vi "BM0211-Image Editing.vi"(8 "error IN":errorcluster) -> (0 "error out":errorcluster)   [LabVIEW 2015]
uses:
  <vilib>/Utility/miscctls.llb/LVBoundsTypeDef.ctl
  <vilib>/Utility/miscctls.llb/LVPointTypeDef.ctl
  Galobal variable_TI.vi
panel:
  in  "Numeric":dbl
  out "2D Picture 2":picture
  out "Assembly ST-1":picture
  out "filenames":string[](array[string])
  out "selected path":path
  out "Boolean":bool
  in  "Vertical position":sgl(slide) min=-2000 max=2000 scale=-1000.0..2000.0 scale format="%#.0f"
  out "Horizontal position":sgl(slide) min=-2000 max=2000 scale=-1000.0..2000.0 scale format="%#.0f"
  in  "Zoom Factor":sgl(slide)=1.0 min=1 max=100 scale=0.0..200.0 scale format="%#.0f"
  out "2D Picture":picture
  in  "Stop Button":bool
  in  "Select Part":u16(ring) items=["P1.JPG", "P2.JPG", "P3.JPG", "P4.JPG", "P5.JPG", "P6.JPG", "P7.JPG", "P8.JPG", "P9.JPG", "P10.JPG", "P11.JPG", "P12.JPG", "P13.JPG", "P14.JPG", "P15.JPG", "P16.JPG", "P17.JPG"]
  in  "Save":bool
  in  "Select New":bool
  # "Image Editing"
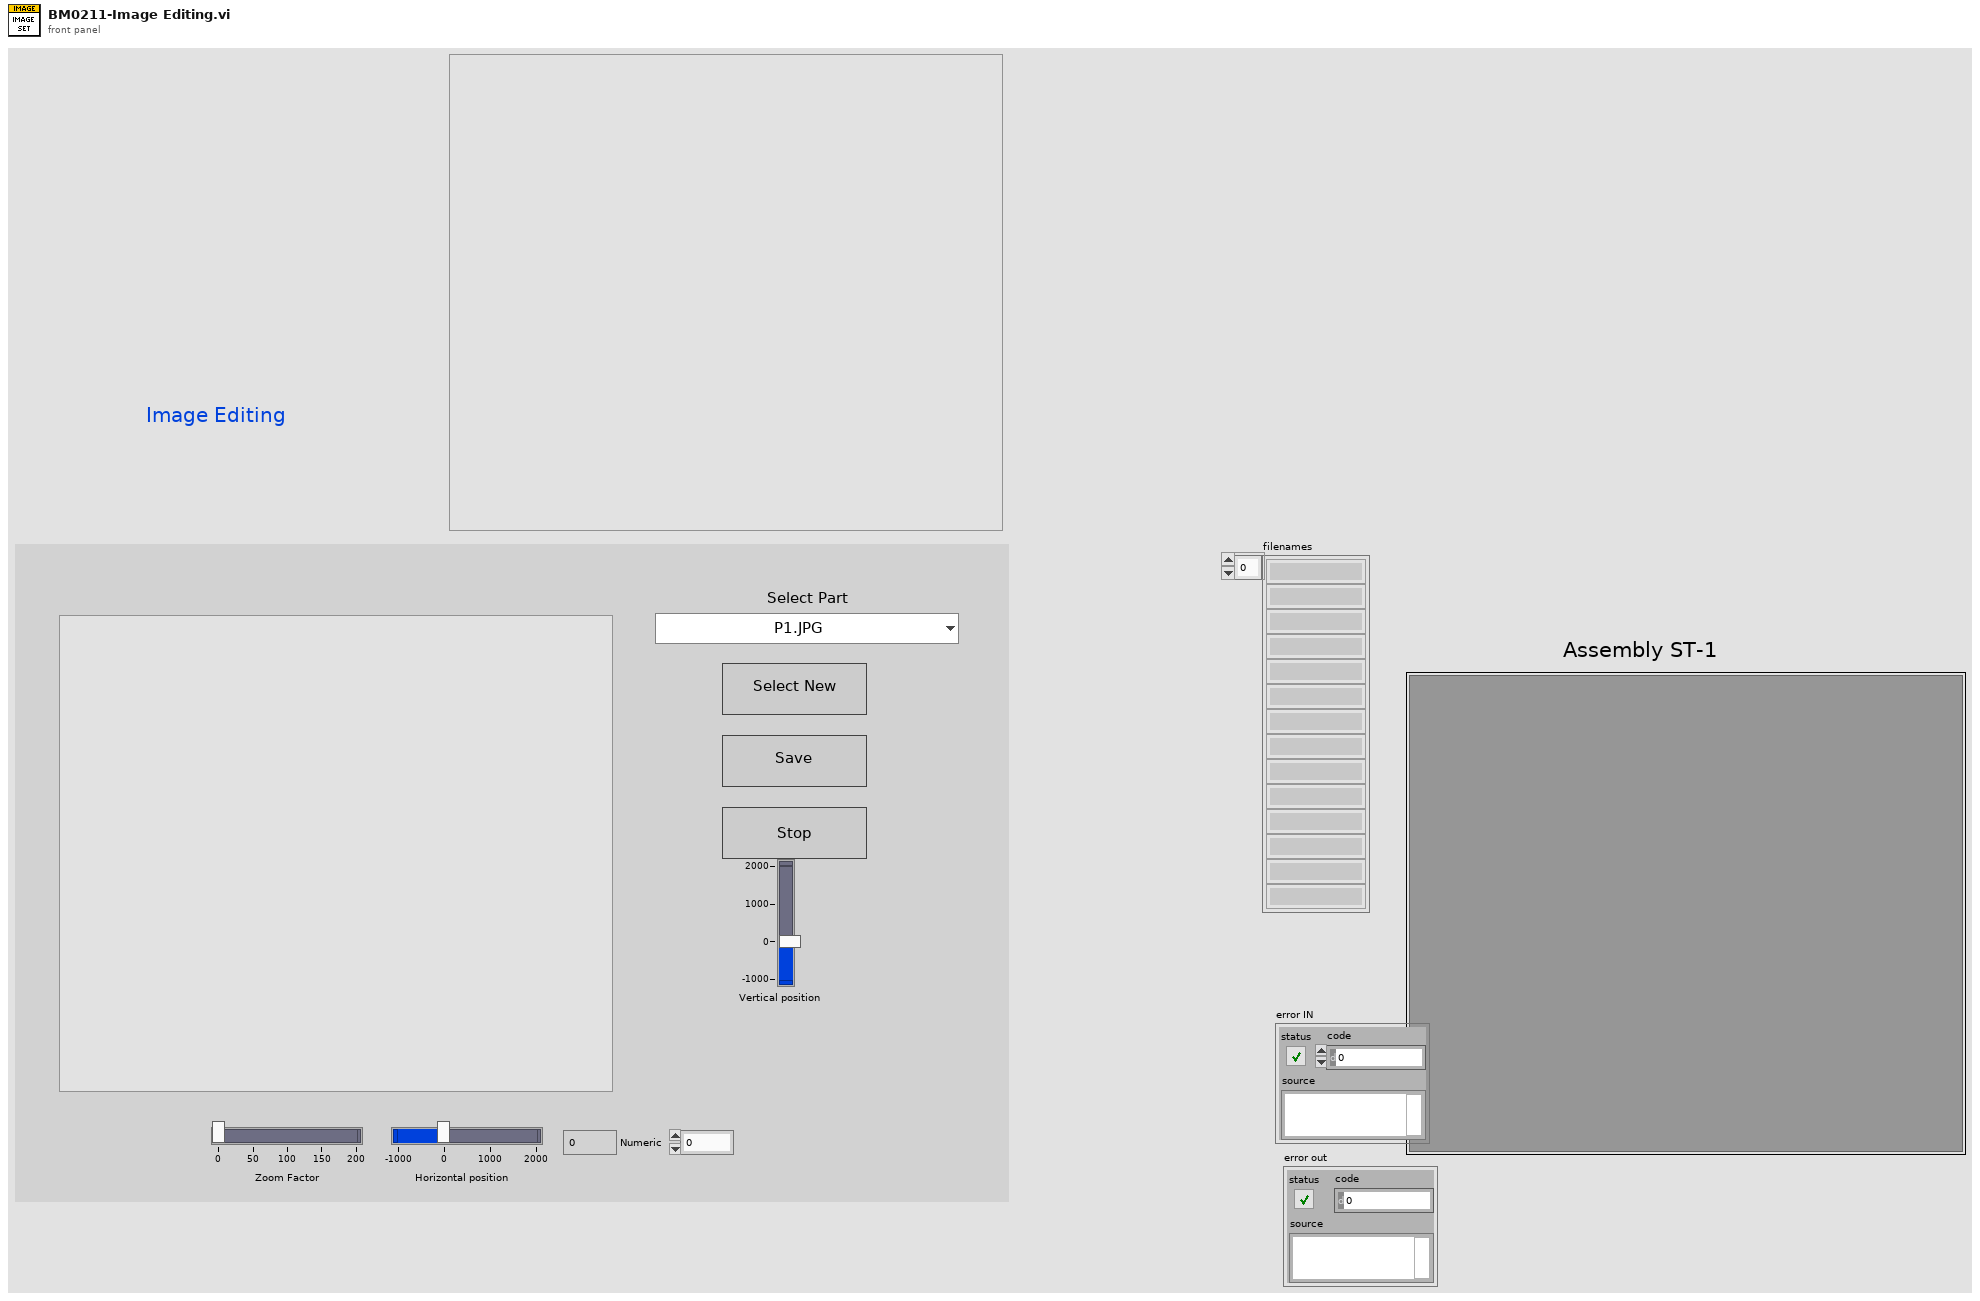
[diagram p1: front panel]
types:
  T1 = typedef "imagedata.ctl" = cluster{"image type":i32, "image depth":i32, "image":u8[], "mask":u8[], "colors":u32[], "Rectangle":cluster{"left":i16, "top":i16, "right":i16, "bottom":i16}}
  T2 = cluster{"Zoom Factor":sgl, "Horizontal position":sgl, "Vertical position":sgl}[]
  T3 = cluster{"Zoom Factor":sgl, "Horizontal position":sgl, "Vertical position":sgl}
  T4 = typedef "LVPointTypeDef.ctl" = cluster{"Horizontal":i16, "Vertical":i16}
  T5 = typedef "LVBoundsTypeDef.ctl" = cluster{"Width":u32, "Height":u32}
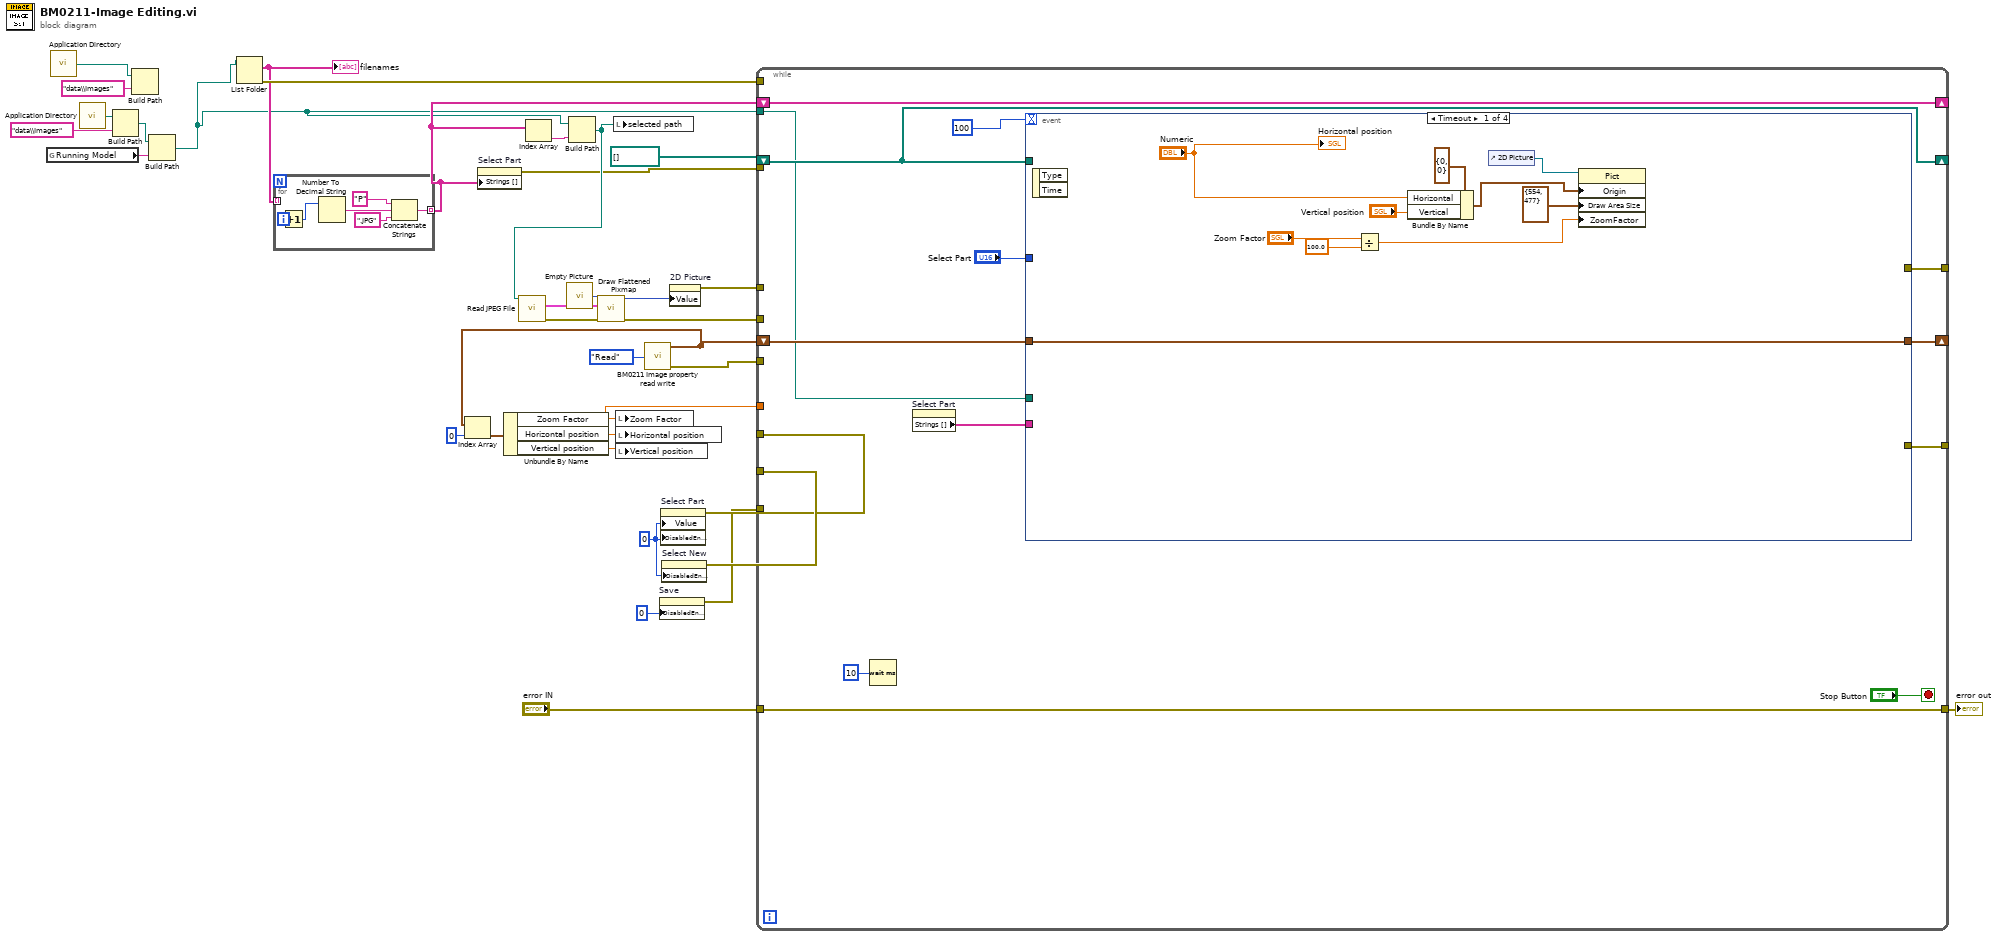
[diagram p0: block diagram]
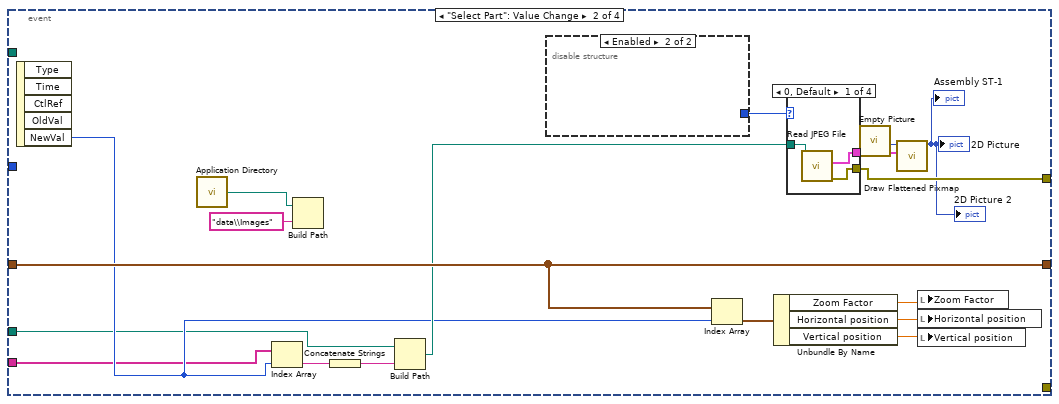
[diagram p2: hidden frame]
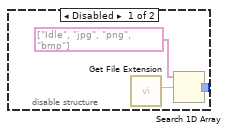
[diagram p3: hidden frame]
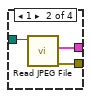
[diagram p4: hidden frame]
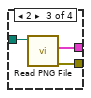
[diagram p5: hidden frame]
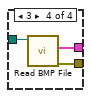
[diagram p6: hidden frame]
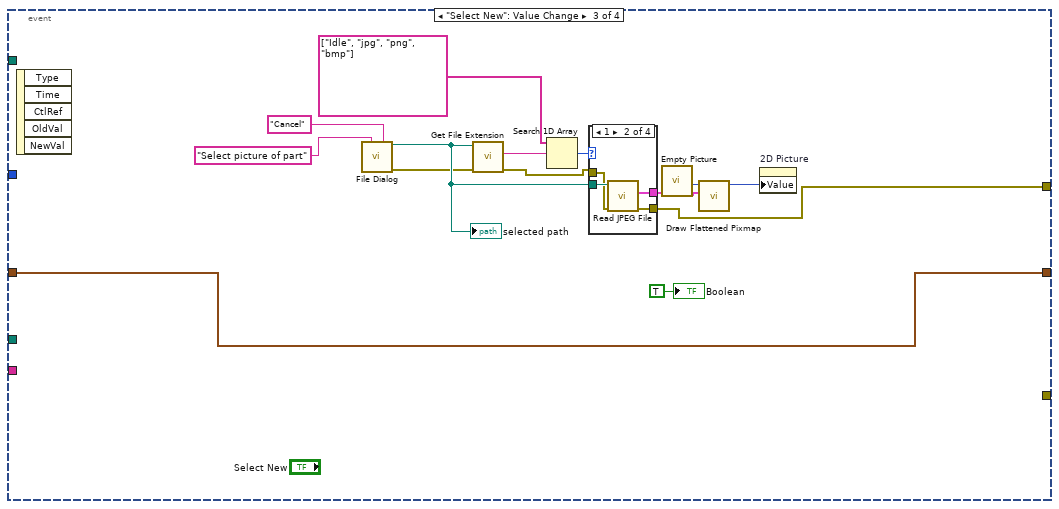
[diagram p7: hidden frame]
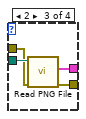
[diagram p9: hidden frame]
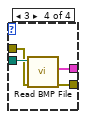
[diagram p10: hidden frame]
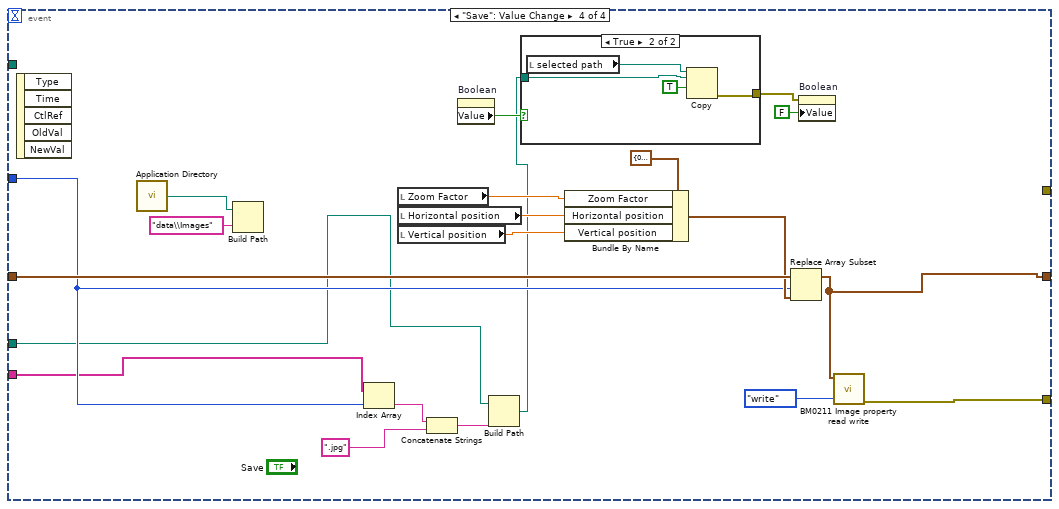
[diagram p11: hidden frame]
diagram:
  w18 = 0
  n1 = global read "Galobal variable_TI.vi" "Running Model"() -> (w2:string)
  n2 = call <vilib>:"Application Directory.vi"() -> ("Application Directory"=w12:path)
  n3 = call <vilib>:"Application Directory.vi"() -> ("Application Directory"=w5:path)
  n4 = Build Path(base path=w5, name or relative path="data\\Images") -> (appended path=w3:path)
  n5 = Build Path(base path=w12, name or relative path="data\\Images") -> ()  [unwired: 1 out]
  n6 = Build Path(base path=w3, name or relative path=w2) -> (appended path=w1:path)
  n7 = List Folder(path=w1) -> (filenames=w7:string[], error out=w17:errorcluster)  [unwired: 3 in, 2 out]
  "filenames" <- w7
  n8 = for {
    tunnel: w7 -> [_] mode=indexing
    tunnel: [w36] -> w6 mode=indexing
    i -> [w40]
    n9 = Increment(x=w40) -> (x+1=w35:i32)
    n10 = Number To Decimal String(number=w35) -> (decimal integer string=w38:string)  [unwired: 1 in]
    n11 = Concatenate Strings("P" ("string"), w38, ".JPG" ("string")) -> (w36:string)
  }
  n12 = property on="Select Part" class="Ring (strict)"("Strings []"=w6) -> (error out=w10:errorcluster)  [unwired: 2 in, 1 out]
  n13 = Index Array(array=w6) -> (element=w16:string)  [unwired: 1 in]
  n14 = call "Empty Picture"() -> ("empty picture"=w24:picture)
  n15 = Build Path(base path=w1, name or relative path=w16) -> (appended path=w13:path)
  n16 = call <vilib>:"Read JPEG File.vi"("path to JPEG file"=w13) -> ("error out"=w22:errorcluster, "image data"=w23:T1)  [unwired: 8 in, 1 out]
  n17 = call <vilib>:"Draw Flattened Pixmap.vi"("image data"=w23, "picture"=w24) -> ("new picture"=w21:picture)  [unwired: 7 in]
  n18 = local write "selected path"(w13) -> ()
  n19 = call "BM0211 Image property read write.vi"("Read write"=enum16{"write", "Read"}."Read") -> ("error out"=w14:errorcluster, "Out"=w27:T2)  [unwired: 9 in]
  n20 = Index Array(array=w27, index=0) -> (element=w28:T3)
  n21 = Unbundle By Name(w28) -> ("Zoom Factor"=w25:sgl, "Horizontal position"=w29:sgl, "Vertical position"=w30:sgl)
  n22 = local write "Zoom Factor"(w25) -> ()
  n23 = local write "Horizontal position"(w29) -> ()
  n24 = local write "Vertical position"(w30) -> ()
  n25 = property on="Save" class="Bool"("DisabledEnum"=0) -> (error out=w31:errorcluster)  [unwired: 2 in, 1 out]
  n26 = property on="Select Part" class="Ring (strict)"("Value"=w18, "DisabledEnum"=w18) -> (error out=w33:errorcluster)  [unwired: 2 in, 1 out]
  n27 = property on="Select New" class="Bool"("DisabledEnum"=w18) -> (error out=w34:errorcluster)  [unwired: 2 in, 1 out]
  n28 = property on="2D Picture" class="Pict"("Value"=w21) -> (error out=w20:errorcluster)  [unwired: 2 in, 1 out]
  n29 = while {
    shift-right: [w51] -> _
    shift-left: path[] [] ("Array") -> [w51]
    tunnel: [w50] -> _
    shift-right: [w47] -> _
    shift-left: w27 -> [w49]
    tunnel: w34 -> [_]
    tunnel: w33 -> [_]
    tunnel: w31 -> [_]
    tunnel: w25 -> [_]
    tunnel: w22 -> [_]
    tunnel: w20 -> [_]
    tunnel: w17 -> [_]
    shift-right: [w45] -> _
    shift-left: w6 -> [w45]
    tunnel: w14 -> [_]
    tunnel: [w44] -> _
    tunnel: w10 -> [_]
    tunnel: "error IN" -> [w42]
    tunnel: [w42] -> w8
    tunnel: w1 -> [w41]
    stop <- "Stop Button" stop-if-true
    n30 = Wait (ms)(milliseconds to wait=u32 10) -> ()  [unwired: 1 out]
    n31 = property on="Select Part" class="Ring (strict)"() -> ("Strings []"=w43:string[])  [unwired: 2 in, 2 out]
    n32 = event shown="[0] Timeout" {
      selector: _ -> [_ _ _ _]
      dyn-events: _ -> [_ _ _ _]
      timeout: 100 -> [_ _ _ _]
      tunnel: w51 -> [_ _ _ _]
      tunnel: [_ w80 w99 _] -> w50
      tunnel: w49 -> [w57 w77 w97 w137]
      tunnel: "Select Part" -> [_ _ _ w134]
      tunnel: [w57 w77 w97 w129] -> w47
      tunnel: [_ _ _ w132] -> w44
      tunnel: w43 -> [_ w66 _ w126]
      tunnel: w41 -> [_ w64 _ w124]
      event Timeout {
        n33 = event-data() -> ()  [unwired: 1 in, 2 out]
        n34 = Divide(x="Zoom Factor", y=sgl 100.0 ("x")) -> (x/y=w55:sgl)
        n35 = Bundle By Name(cluster=T4 {"Horizontal"=0, "Vertical"=0} ("Origin"), "Horizontal"="Numeric", "Vertical"="Vertical position") -> (w56:T4)
        n36 = control-ref of="2D Picture"() -> (w61:refnum<vi>)
        n37 = property class="Pict"(reference=w61, "Origin"=w56, "Draw Area Size"=T5 {"Width"=554, "Height"=477}, "ZoomFactor"=w55) -> ()  [unwired: 1 in, 2 out]
        "Horizontal position" <- "Numeric"
      }
      event "Select Part": Value Change {
        n38 = event-data() -> ("NewVal"=w69:u16)  [unwired: 1 in, 4 out]
        n39 = call <vilib>:"Application Directory.vi"() -> ("Application Directory"=w68:path)
        n40 = Index Array(array=w66, index=w69) -> (element=w72:string)
        n41 = Build Path(base path=w68, name or relative path="data\\Images") -> ()  [unwired: 1 out]
        n42 = Concatenate Strings(w72) -> (w70:string)
        n43 = Build Path(base path=w64, name or relative path=w70) -> (appended path=w71:path)
        n44 = disable-structure shown="Enabled" {
          disable-tunnel: [w82 _] -> w79
          frame Disabled {
            n45 = call <vilib>:"Get File Extension.vi"() -> ("lowercase file extension"=w83:string)  [unwired: 7 in, 4 out]
            n46 = Search 1D Array(1D array=string[] ["Idle", "jpg", "png", "bmp"] ("Strings []"), element=w83) -> (index of element=w82:i32)  [unwired: 1 in]
          }
          frame Enabled {
          }
        }
        n47 = Index Array(array=w77, index=w69) -> (element=w76:T3)
        n48 = Unbundle By Name(w76) -> ("Zoom Factor"=w75:sgl, "Horizontal position"=w74:sgl, "Vertical position"=w73:sgl)
        n49 = case shown="0, Default" w79 {
          tunnel: [w86 w90 w92 w95] -> w78
          tunnel: [w85 w89 w91 w96] -> w80
          tunnel: w71 -> [w87 w88 w93 w94]
          frame 0, Default {
            n50 = call <vilib>:"Read JPEG File.vi"("path to JPEG file"=w87) -> ("error out"=w85:errorcluster, "image data"=w86:T1)  [unwired: 8 in, 1 out]
          }
          frame 1 {
            n51 = call <vilib>:"Read JPEG File.vi"("path to JPEG file"=w88) -> ("error out"=w89:errorcluster, "image data"=w90:T1)  [unwired: 8 in, 1 out]
          }
          frame 2 {
            n52 = call <vilib>:"Read PNG File.vi"("path to PNG file"=w93) -> ("error out"=w91:errorcluster, "image data"=w92:T1)  [unwired: 8 in, 1 out]
          }
          frame 3 {
            n53 = call <vilib>:"Read BMP File.vi"("path to BMP file"=w94) -> ("error out"=w96:errorcluster, "image data"=w95:T1)  [unwired: 8 in, 1 out]
          }
        }
        n54 = call "Empty Picture"() -> ("empty picture"=w81:picture)
        n55 = call <vilib>:"Draw Flattened Pixmap.vi"("image data"=w78, "picture"=w81) -> ("new picture"=→"2D Picture" →"Assembly ST-1" →"2D Picture 2":picture)  [unwired: 7 in]
        n56 = local write "Zoom Factor"(w75) -> ()
        n57 = local write "Horizontal position"(w74) -> ()
        n58 = local write "Vertical position"(w73) -> ()
      }
      event "Select New": Value Change {
        n59 = event-data() -> ()  [unwired: 1 in, 5 out]
        n60 = call "File Dialog"("prompt"="Select picture of part", "button label"="Cancel") -> ("selected path"=w102:path, "error out"=w101:errorcluster)  [unwired: 10 in, 2 out]
        "selected path" <- w102
        n61 = call <vilib>:"Get File Extension.vi"("error in (no error)"=w101, "file"=w102) -> ("error out"=w106:errorcluster, "lowercase file extension"=w108:string)  [unwired: 5 in, 3 out]
        n62 = Search 1D Array(1D array=string[] ["Idle", "jpg", "png", "bmp"] ("Strings []"), element=w108) -> (index of element=w107:i32)  [unwired: 1 in]
        n63 = case shown="1" w107 {
          tunnel: [_ w115 w119 w122] -> w100
          tunnel: [w111 w114 w118 w123] -> w99
          tunnel: w106 -> [w111 w112 w116 w120]
          tunnel: w102 -> [_ w113 w117 w121]
          frame 0, Default {
          }
          frame 1 {
            n64 = call <vilib>:"Read JPEG File.vi"("error in (no error)"=w112, "path to JPEG file"=w113) -> ("error out"=w114:errorcluster, "image data"=w115:T1)  [unwired: 7 in, 1 out]
          }
          frame 2 {
            n65 = call <vilib>:"Read PNG File.vi"("error in (no error)"=w116, "path to PNG file"=w117) -> ("error out"=w118:errorcluster, "image data"=w119:T1)  [unwired: 7 in, 1 out]
          }
          frame 3 {
            n66 = call <vilib>:"Read BMP File.vi"("error in (no error)"=w120, "path to BMP file"=w121) -> ("error out"=w123:errorcluster, "image data"=w122:T1)  [unwired: 7 in, 1 out]
          }
        }
        n67 = call "Empty Picture"() -> ("empty picture"=w110:picture)
        n68 = call <vilib>:"Draw Flattened Pixmap.vi"("image data"=w100, "picture"=w110) -> ("new picture"=w105:picture)  [unwired: 7 in]
        n69 = property on="2D Picture" class="Pict"("Value"=w105) -> ()  [unwired: 2 in, 2 out]
        "Boolean" <- TRUE
      }
      event "Save": Value Change {
        n70 = event-data() -> ()  [unwired: 1 in, 5 out]
        n71 = call <vilib>:"Application Directory.vi"() -> ("Application Directory"=w128:path)
        n72 = Build Path(base path=w128, name or relative path="data\\Images") -> ()  [unwired: 1 out]
        n73 = Index Array(array=w126, index=w134) -> (element=w125:string)
        n74 = local read "Zoom Factor"() -> (w141:sgl)
        n75 = local read "Horizontal position"() -> (w140:sgl)
        n76 = local read "Vertical position"() -> (w139:sgl)
        n77 = Concatenate Strings(w125, ".jpg" ("string")) -> (w131:string)
        n78 = property on="Boolean" class="Bool (strict)"() -> ("Value"=w144:bool)  [unwired: 2 in, 2 out]
        n79 = Build Path(base path=w124, name or relative path=w131) -> (appended path=w133:path)
        n80 = case shown="True" w144 {
          tunnel: w133 -> [_ w145]
          tunnel: [_ w148] -> w142
          frame False {
          }
          frame True {
            n81 = local read "selected path"() -> (w147:path)
            n82 = Copy(9:TRUE ("overwrite (F)"), 10:w145, 11:w147) -> (0:w148:errorcluster)  [unwired: 2 in, 2 out]
          }
        }
        n83 = Bundle By Name(cluster=T3 {"Zoom Factor"=0.0, "Horizontal position"=0.0, "Vertical position"=0.0} ("element"), "Zoom Factor"=w141, "Horizontal position"=w140, "Vertical position"=w139) -> (w136:T3)
        n84 = Replace Array Subset(array=w137, new element=w136, index=w134) -> (w129:T2)
        n85 = property on="Boolean" class="Bool (strict)"(error in=w142, "Value"=FALSE ("Boolean")) -> ()  [unwired: 1 in, 2 out]
        n86 = call "BM0211 Image property read write.vi"("Read write"=enum16{"write", "Read"}."write", "IN"=w129) -> ("error out"=w132:errorcluster)  [unwired: 8 in, 1 out]
      }
    }
  }
  "error out" <- w8
